vi "ReadLeonardoJoystick.vi"(8 "error in (no error)":errorcluster, 10 "Previous buttons":bool[](array[boolean]), 11 "Refnum in":refnum<k1>) -> (0 "error out":errorcluster, 2 "buttons":bool[](array[boolean]), 3 "Refnum out":refnum<k1>)   [LabVIEW 2014]
doc: "Red button states from Arduino. On error, reinitialize connection and return previous state"
uses:
  <vilib>/Utility/inputDevices.llb/joystickAcquire.vi
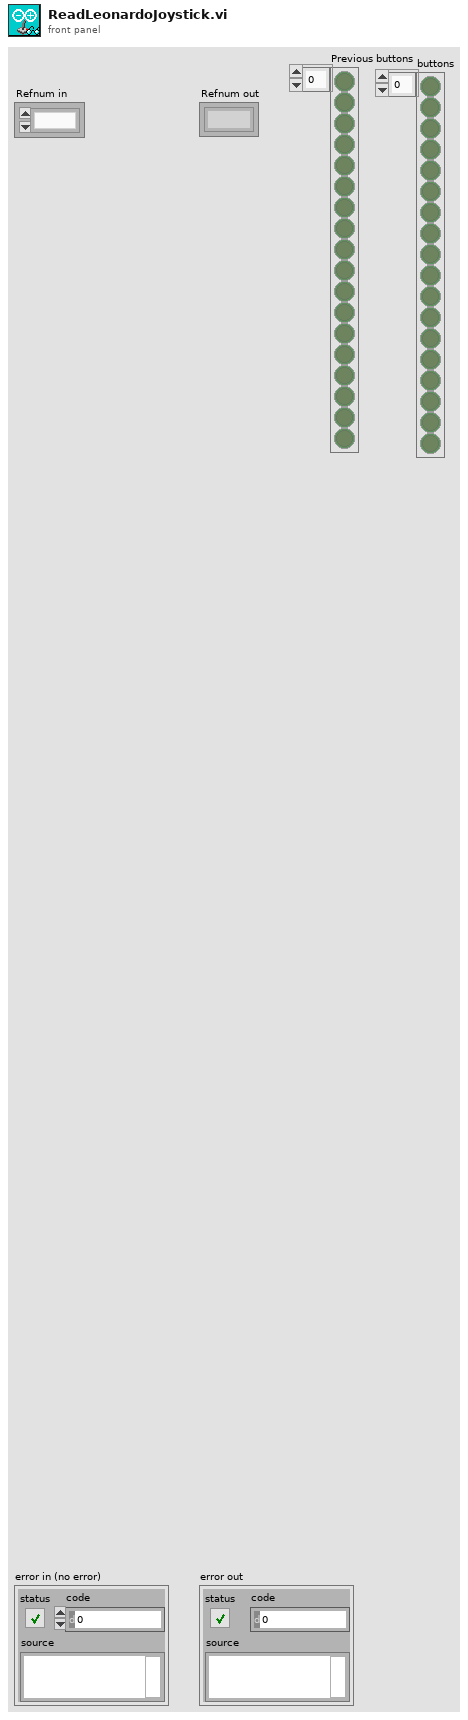
[diagram p1: front panel]
types:
  T1 = cluster{"button 1":bool, "button 2":bool, "button 3":bool, "button 4":bool, "button 5":bool, "button 6":bool, "button 7":bool, "button 8":bool, "button 9":bool, "button 10":bool, "button 11":bool, "button 12":bool, "button 13":bool, "button 14":bool, "button 15":bool, "button 16":bool, "button 17":bool, "button 18":bool, "button 19":bool, "button 20":bool, "button 21":bool, "button 22":bool, "button 23":bool, "button 24":bool, "button 25":bool, "button 26":bool, "button 27":bool, "button 28":bool, "button 29":bool, "button 30":bool, "button 31":bool, "button 32":bool}
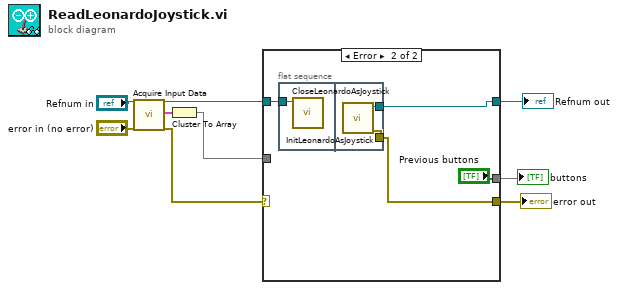
[diagram p0: block diagram]
diagram:
  n1 = call-poly <vilib>:"Acquire Input Data.vi"("device ID"="Refnum in", "error in (no error)"="error in (no error)") -> ("device ID"=w2:refnum<k1>, "button info"=w7:T1, "error out"=w6:errorcluster)  [unwired: 13 in, 2 out]
  n2 = Cluster To Array(cluster=w7) -> (array=w4:bool[])
  n3 = case shown="Error" w6 {
    selector: w6 -> [w12 _]
    tunnel: [w12 w15] -> w5
    tunnel: w4 -> [w11 _]
    tunnel: [w11 "Previous buttons"] -> w3
    tunnel: w2 -> [w10 w13]
    tunnel: [w10 w16] -> w1
    frame No Error {
    }
    frame Error {
      n4 = flat-sequence {
        tunnel: w13 -> [w17]
        tunnel: [w19] -> w16
        tunnel: [w18] -> w15
        frame #0 {
          n5 = call "CloseLeonardoAsJoystick.vi"("Refnum in"=w17) -> ()  [unwired: 11 in]
        }
        frame #1 {
          n6 = call "InitLeonardoAsJoystick.vi"() -> ("error out"=w18:errorcluster, "Refnum out"=w19:refnum<k1>)  [unwired: 10 in]
        }
      }
    }
  }
  "error out" <- w5
  "Refnum out" <- w1
  "buttons" <- w3
